vi "DAQ_SaveParams.vi"(11 "Params":T1) -> (0 "error out":errorcluster)   [LabVIEW 2019]
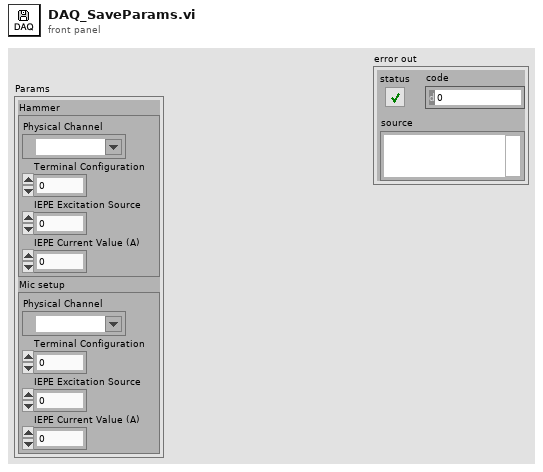
[diagram p1: front panel]
types:
  T1 = cluster{"Hammer":cluster{"Physical Channel":tag, "Terminal Configuration":i32, "IEPE Excitation Source":i32, "IEPE Current Value (A)":dbl}, "Mic setup":cluster{"Physical Channel":tag, "Terminal Configuration":i32, "IEPE Excitation Source":i32, "IEPE Current Value (A)":dbl}}
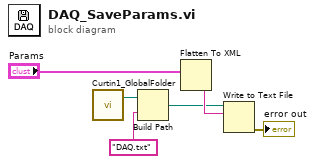
[diagram p0: block diagram]
diagram:
  n1 = call "Curtin1_GlobalFolder.vi"() -> ("LabVIEW Data Path"=w3:path)  [unwired: 1 in, 1 out]
  n2 = Build Path(base path=w3, name or relative path="DAQ.txt") -> (appended path=w2:path)
  n3 = Flatten To XML(anything="Params") -> (xml string=w4:string)
  n4 = Write to Text File(file (use dialog)=w2, text=w4) -> (error out=→"error out":errorcluster)  [unwired: 2 in, 2 out]
